vi "Normatização.vi"(8 "error in (no error)":errorcluster, 9 "Amplitude Refnum":refnum<vi>, 10 "Offset Refnum":refnum<vi>, 11 "Cluster":T1={"Estados"=enum."Gerar onda", "Amplitude"=0.0, "Informação\nde amostragem"={"Fs"=1000.0, "#s"=1000.0}, "Frequência"=0.0, "Offset"=0.0, "Fase (Graus)"=0.0, "Razão cíclica (%)"=0.0, "Sinal"=enum."Sine Wave"}) -> (0 "error out":errorcluster, 3 "Cluster":T1={"Estados"=enum."Gerar onda", "Amplitude"=0.0, "Informação\nde amostragem"={"Fs"=1000.0, "#s"=1000.0}, "Frequência"=0.0, "Offset"=0.0, "Fase (Graus)"=0.0, "Razão cíclica (%)"=0.0, "Sinal"=enum."Sine Wave"})   [LabVIEW 2019]
uses:
  Estados - Consumidor.ctl
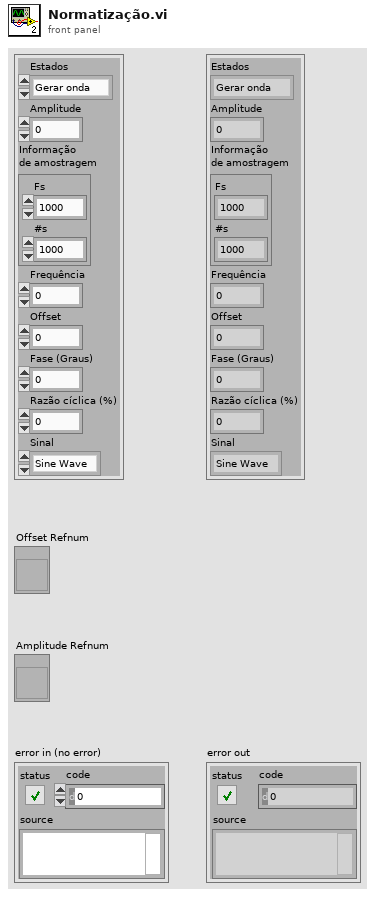
[diagram p1: front panel]
types:
  T1 = typedef "Informações.ctl" = cluster{"Estados":T2, "Amplitude":dbl, "Informação\nde amostragem":cluster{"Fs":dbl, "#s":dbl}, "Frequência":dbl, "Offset":dbl, "Fase (Graus)":dbl, "Razão cíclica (%)":dbl, "Sinal":enum16{"Sine Wave", "Triangle Wave", "Square Wave", "Sawtooth Wave", "Trapezoidal Wave"}}
  T2 = typedef "Estados - Consumidor.ctl" = enum16{"Gerar onda", "Inicialização", "Parada", "Plotar", "Concatenar", "Concatenar - Cursores", "Adquirir entre Cursores", "Deletar entre Cursores", "Salvar onda", "Carregar onda"}
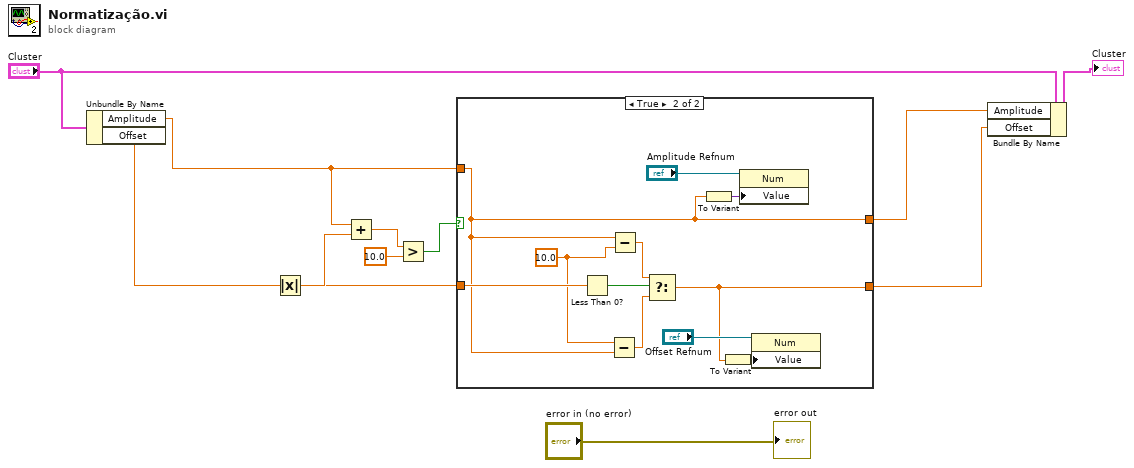
[diagram p0: block diagram]
diagram:
  n1 = Unbundle By Name("Cluster") -> ("Amplitude"=w5:dbl, "Offset"=w4:dbl)
  n2 = Absolute Value(x=w4) -> (abs(x)=w8:dbl)
  n3 = Add(x=w5, y=w8) -> (x+y=w10:dbl)
  n4 = Greater?(x=w10, y=10.0) -> (0:w9:bool)
  n5 = case shown="True" w9 {
    tunnel: w5 -> [w13 w15]
    tunnel: w4 -> [w12 w24]
    tunnel: [w13 w15] -> w3
    tunnel: [w12 w18] -> w2
    frame False {
    }
    frame True {
      w20 = 10.0 ("y")
      n6 = Less Than 0?(x=w24) -> (x < 0?=w23:bool)
      n7 = Subtract(x=w20, y=w15) -> (x-y=w22:dbl)
      n8 = Subtract(x=w15, y=w20) -> (x-y=w21:dbl)
      n9 = Select(t=w21, s=w23, f=w22) -> (s? t:f=w18:dbl)
      n10 = To Variant(anything=w15) -> (Variant=w16:variant)
      n11 = To Variant(anything=w18) -> (Variant=w14:variant)
      n12 = property class="Num"(reference="Amplitude Refnum", "Value"=w16) -> ()  [unwired: 1 in, 2 out]
      n13 = property class="Num"(reference="Offset Refnum", "Value"=w14) -> ()  [unwired: 1 in, 2 out]
    }
  }
  n14 = Bundle By Name(cluster="Cluster", "Amplitude"=w3, "Offset"=w2) -> (→"Cluster":T1)
  "error out" <- "error in (no error)"
